vi "Add New State.vi"(8 "error in (no error)":errorcluster, 9 "State Name":string, 10 "Category (Optional)":string, 11 "JKI SM in":refnum<class "JKI SM.lvclass">) -> (0 "error out":errorcluster, 1 "New Frame Index":i32, 3 "JKI SM out":refnum<class "JKI SM.lvclass">)   [LabVIEW 2013, in "JKI State Machine API.lvlib" / "JKI SM.lvclass"]
uses:
  JKI SM.lvclass
  JKI SM.lvclass/JKI SM.ctl
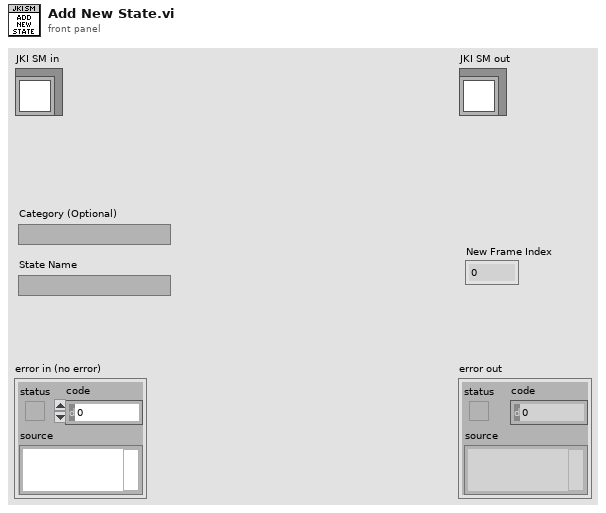
[diagram p1: front panel]
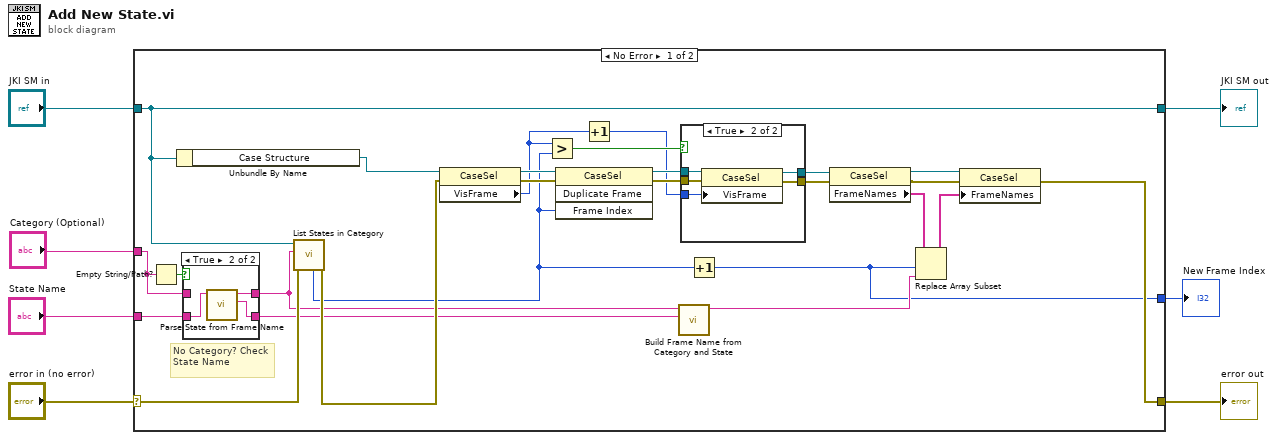
[diagram p0: block diagram]
diagram:
  n1 = case shown="No Error" "error in (no error)" {
    selector: "error in (no error)" -> [w28 w47]
    tunnel: [w27 w47] -> w6
    tunnel: [w33 w46] -> w4
    tunnel: "JKI SM in" -> [w33 w46]
    tunnel: "State Name" -> [w11 _]
    tunnel: "Category (Optional)" -> [w12 _]
    tunnel: [w8 _] -> w1
    frame No Error {
      # "No Category? Check State Name"
      n2 = Empty String/Path?(string/path=w12) -> (empty?=w14:bool)
      n3 = Unbundle By Name(w33) -> ("Case Structure"=w25:refnum<vi>)
      n4 = case shown="True" w14 {
        tunnel: w11 -> [w34 w38]
        tunnel: [w35 w37] -> w13
        tunnel: w12 -> [w35 _]
        tunnel: [w34 w36] -> w10
        frame False {
        }
        frame True {
          n5 = call "Parse State from Frame Name.vi"("Frame Name"=w38) -> ("State Name"=w36:string, "Category Name"=w37:string)  [unwired: 7 in, 2 out]
        }
      }
      n6 = call "List States in Category.vi"("error in (no error)"=w28, "Category"=w13, "JKI SM in"=w33) -> ("error out"=w23:errorcluster, "Category Frame Index"=w9:i32)  [unwired: 4 in, 3 out]
      n7 = property class="CaseSel"(reference=w25, error in=w23) -> (reference out=w24:refnum<vi>, error out=w22:errorcluster, "VisFrame"=w17:u32)
      n8 = Greater?(x=w17, y=w9) -> (0:w16:bool)
      n9 = invoke class="CaseSel" method="Duplicate Frame"(reference=w24, error in=w22, "Frame Index"=w9) -> (reference out=w19:refnum<vi>, error out=w18:errorcluster)  [unwired: 1 in, 2 out]
      n10 = Increment(x=w17) -> (x+1=w15:u32)
      n11 = call "Build Frame Name from Category and State.vi"("State Name"=w10, "Category"=w13) -> ("Frame Name"=w26:string)  [unwired: 9 in]
      n12 = case shown="True" w16 {
        tunnel: [w40 w45] -> w21
        tunnel: [w39 w44] -> w20
        tunnel: w19 -> [w40 w43]
        tunnel: w18 -> [w39 w42]
        tunnel: w15 -> [_ w41]
        frame False {
        }
        frame True {
          n13 = property class="CaseSel"(reference=w43, error in=w42, "VisFrame"=w41) -> (reference out=w45:refnum<vi>, error out=w44:errorcluster)
        }
      }
      n14 = Increment(x=w9) -> (x+1=w8:i32)
      n15 = property class="CaseSel"(reference=w21, error in=w20) -> (reference out=w32:refnum<vi>, error out=w31:errorcluster, "FrameNames"=w30:string[])
      n16 = Replace Array Subset(array=w30, new element=w26, index=w8) -> (w29:string[])
      n17 = property class="CaseSel"(reference=w32, error in=w31, "FrameNames"=w29) -> (error out=w27:errorcluster)  [unwired: 1 out]
    }
    frame Error {
    }
  }
  "error out" <- w6
  "JKI SM out" <- w4
  "New Frame Index" <- w1
